vi "ReadWrite.ProcessData.Write.vi"(7 "error in (no error)":errorcluster, 8 "Offset":i32, 9 "Values":dbl[](array[numeric]), 10 "ReadWrite in":refnum<class "ReadWrite.lvclass">) -> (0 "error out":errorcluster, 3 "ReadWrite out":refnum<class "ReadWrite.lvclass">)   [LabVIEW 2015, in "Data Access Engine.lvlib" / "ReadWrite.lvclass"]
uses:
  ReadWrite.lvclass
  ReadWrite.lvclass/ReadWrite.ctl
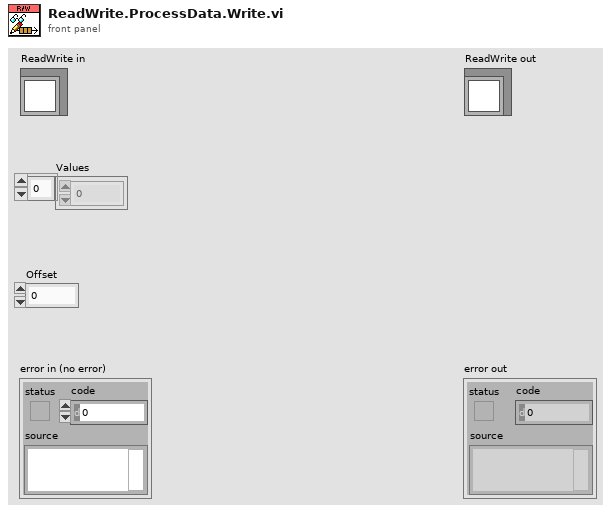
[diagram p1: front panel]
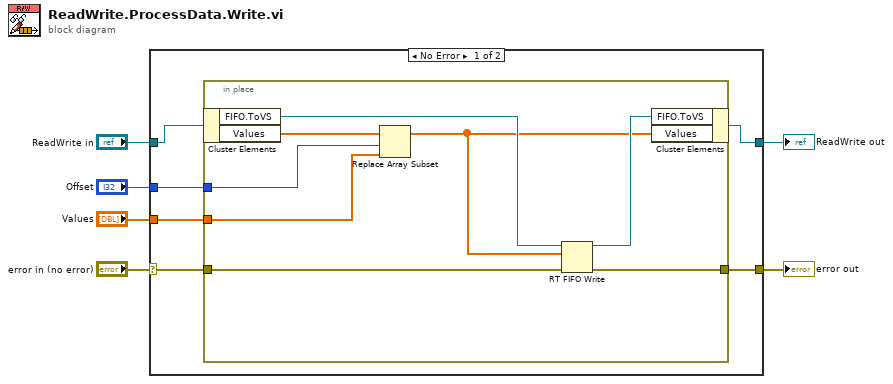
[diagram p0: block diagram]
diagram:
  n1 = case shown="No Error" "error in (no error)" {
    selector: "error in (no error)" -> [w12 w22]
    tunnel: [w11 w22] -> w5
    tunnel: [w9 w21] -> w3
    tunnel: "ReadWrite in" -> [w10 w21]
    tunnel: "Values" -> [w8 _]
    tunnel: "Offset" -> [w7 _]
    frame No Error {
      n2 = in-place {
        in-place-border: w12 -> [w17]
        in-place-border: [w18] -> w11
        in-place-border: w8 -> [w16]
        in-place-border: w7 -> [w14]
        n3 = in-place-cluster #1(w10) -> ("FIFO.ToVS"=w20:refnum<k33>, "Values"=w15:dbl[])
        n4 = Replace Array Subset(array=w15, new element=w16, index=w14) -> (w13:dbl[])
        n5 = RT FIFO Write(0:w20, 1:w13, 3:w17) -> (8:w19:refnum<k33>, 11:w18:errorcluster)  [unwired: 2 in, 2 out]
        n6 = in-place-cluster #1("FIFO.ToVS"=w19, "Values"=w13) -> (w9:refnum<class "ReadWrite.lvclass">)
      }
    }
    frame Error {
    }
  }
  "error out" <- w5
  "ReadWrite out" <- w3
